vi "Run Test (VIRefnum Array).vi"(5 "Test Report":refnum<class "Test Report.lvclass">, 6 "Verbose":bool, 7 "Report Path":path, 8 "error in":errorcluster, 9 "Inspect Recursively (T)":bool=TRUE, 10 "VI Refnums":refnum<vi>[](array[refnum]), 11 "Interactive (T)":bool=TRUE) -> (0 "error out":errorcluster)   [LabVIEW 2013, in "Caraya.lvlib"]
uses:
  Caraya.lvlib
  classes/Test Report/Test Report.lvclass
  classes/Test Runner/Test Runner.lvclass
  classes/Test Runner.Folder/Test Runner.Folder.lvclass
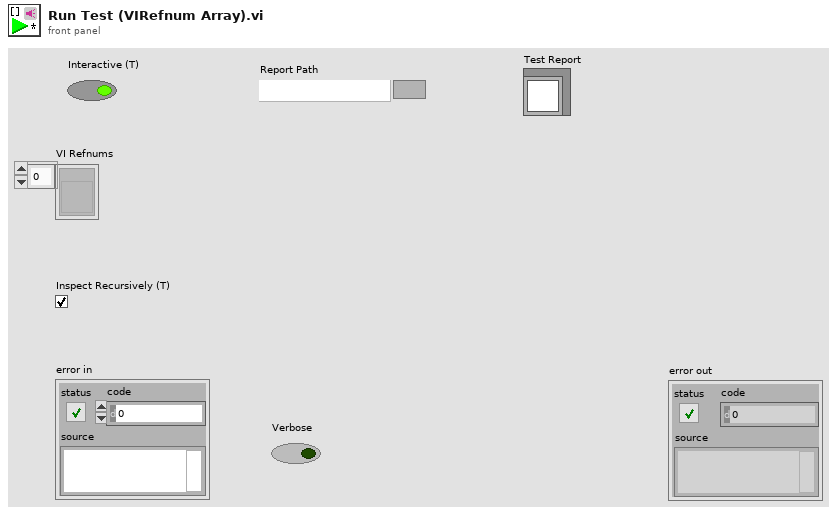
[diagram p1: front panel]
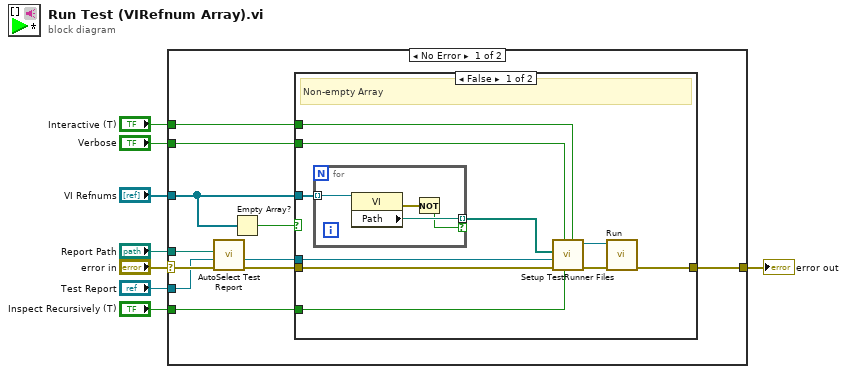
[diagram p0: block diagram]
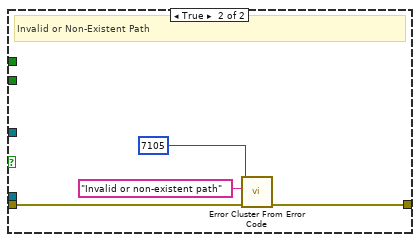
[diagram p2: hidden frame]
diagram:
  n1 = case shown="No Error" "error in" {
    selector: "error in" -> [w16 w38]
    tunnel: [w19 w38] -> w8
    tunnel: "Verbose" -> [w18 _]
    tunnel: "Interactive (T)" -> [w17 _]
    tunnel: "Test Report" -> [w13 _]
    tunnel: "VI Refnums" -> [w10 _]
    tunnel: "Report Path" -> [w15 _]
    tunnel: "Inspect Recursively (T)" -> [w11 _]
    frame No Error {
      n2 = call "AutoSelect Test Report.vi"("error in (no error)"=w16, "Test Report in"=w13, "Report Path"=w15) -> ("error out"=w14:errorcluster, "Test Report out"=w12:refnum<class "Test Report.lvclass">)  [unwired: 7 in]
      n3 = Empty Array?(array=w10) -> (empty?=w9:bool)
      n4 = case shown="False" w9 {
        tunnel: [w29 w36] -> w19
        tunnel: w18 -> [w27 _]
        tunnel: w17 -> [w26 _]
        tunnel: w14 -> [w20 w37]
        tunnel: w12 -> [w24 _]
        tunnel: w11 -> [w23 _]
        tunnel: w10 -> [w22 _]
        frame False {
          # "Non-empty Array"
          n5 = for {
            tunnel: [w33] -> w21 mode=indexing if=w30
            tunnel: w22 -> [w32] mode=indexing
            n6 = property class="VI"(reference=w32) -> (error out=w31:errorcluster, "Path"=w33:path)  [unwired: 1 in, 1 out]
            n7 = Not(x=w31) -> (.not. x?=w30:bool)
          }
          n8 = call "Setup TestRunner Files.vi"("Interactive (T)"=w26, "Inspect Recursively (T)"=w23, "Verbose (F)"=w27, "error in (no error)"=w20, "Test Report"=w24, "Paths"=w21) -> ("error out"=w28:errorcluster, "Test Runner.Folder out"=w25:refnum<class "Test Runner.Folder.lvclass">)  [unwired: 4 in]
          n9 = call "Run.vi"("error in (no error)"=w28, "Test Runner in"=w25) -> ("error out"=w29:errorcluster)  [unwired: 8 in, 1 out]
        }
        frame True {
          # "Invalid or Non-Existent Path"
          n10 = call <vilib>:"Error Cluster From Error Code.vi"("error in (no error)"=w37, "error message (\"\")"="Invalid or non-existent path" ("error message (\"\")"), "error code (0)"=7105 ("code")) -> ("error out"=w36:errorcluster)  [unwired: 6 in]
        }
      }
    }
    frame Error {
    }
  }
  "error out" <- w8
